vi "CryoServer Parse Telemetry JSON.vi"(8 "error in (no error)":errorcluster, 11 "Telemetry String":string) -> (0 "error out":errorcluster, 1 "Timestamp":timestamp, 2 "Values":dbl[](array[numeric]), 3 "Ch Names":string[](array[string]), 4 "Board":string)   [LabVIEW 2024, in "CryoServer.lvclass"]
uses:
  CryoServer.lvclass
  <vilib>/JDP Science/JSONtext/JSONtext.lvlib
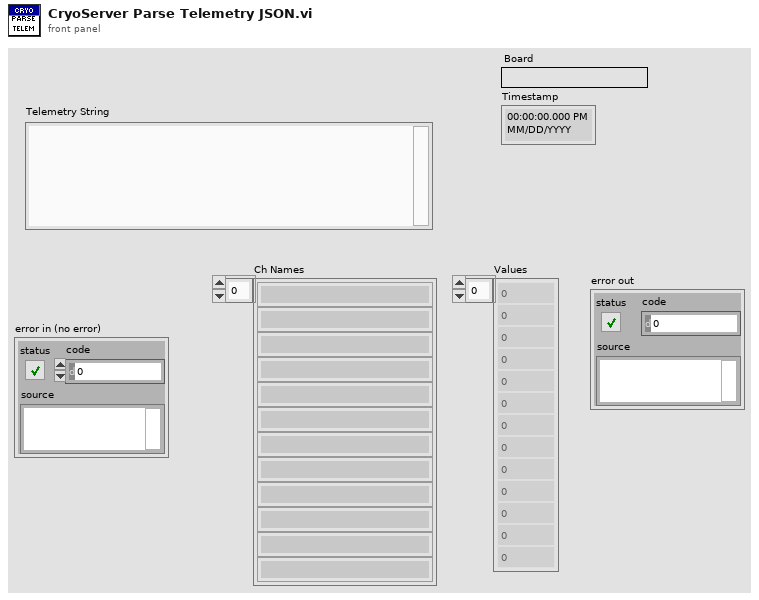
[diagram p1: front panel]
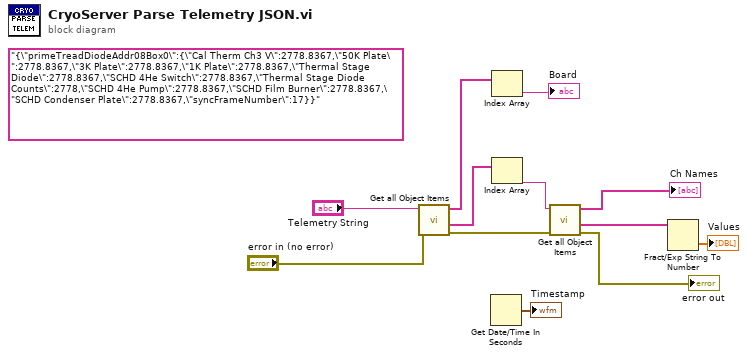
[diagram p0: block diagram]
diagram:
  (unwired) "{\"primeTreadDiodeAddr08Box0\":{\"Cal Therm Ch3 V\":2778.8367,\"50K Plate\":2778.8367,\"3K Plate\":2778.8367,\"1K Plate\":2778.8367,\"Thermal Stage Diode\":2778.8367,\"SCHD 4He Switch\":2778.8367,\"Thermal Stage Diode Counts\":2778,\"SCHD 4He Pump\":2778.8367,\"SCHD Film Burner\":2778.8367,\"SCHD Condenser Plate\":2778.8367,\"syncFrameNumber\":17}}"
  n1 = call <vilib>:"Get all Object Items.vi"("error in (no error)"="error in (no error)", "JSON"="Telemetry String") -> ("error out"=w2:errorcluster, "<JSON>"=w12:string[], "Item Names"=w6:string[])  [unwired: 6 in, 1 out]
  n2 = Get Date/Time In Seconds() -> (seconds since 1Jan1904=→"Timestamp":timestamp)
  n3 = Index Array(array=w6) -> (element=→"Board":string)  [unwired: 1 in]
  n4 = Index Array(array=w12) -> (element=w10:string)  [unwired: 1 in]
  n5 = call <vilib>:"Get all Object Items.vi"("error in (no error)"=w2, "JSON"=w10) -> ("error out"=→"error out":errorcluster, "<JSON>"=w11:string[], "Item Names"=→"Ch Names":string[])  [unwired: 6 in, 1 out]
  n6 = Fract/Exp String To Number(string=w11) -> (number=→"Values":dbl[])  [unwired: 3 in, 1 out]
